vi "float_to_boolean.vi"(11 "Numeric":dbl) -> (3 "Boolean":bool)   [LabVIEW 2019]
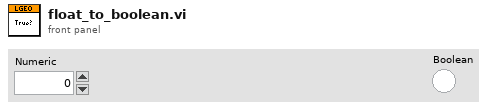
[diagram p1: front panel]
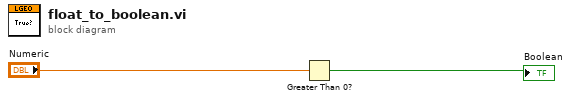
[diagram p0: block diagram]
diagram:
  n1 = Greater Than 0?(x="Numeric") -> (x > 0?=→"Boolean":bool)
